vi "Find Version of Installed Driver 2012 NIVerified.vi"() -> ()   [LabVIEW 2012]
uses:
  <vilib>/nisyscfg/Get Installed Components.vi
  <vilib>/nisyscfg/Close (System).vi
  <vilib>/nisyscfg/nisyscfg.lvlib
panel:
  out "NI-IMAQdx version":string
  out "NI-Serial version":string
  # "Overview: This example demonstrates a method of programmatically getting the version of the NI Software, Drivers, and or Devices by utilizing the System Configuration API.\nRequirements: \n1. LabVIEW 2012 ( or compatible)\n2. NI System Configuration 5.3.3 (or compatible)\nInstructions: \n1. Configure which drivers you would like to find the driver version in the block diagram in the two string constants (This example uses NI-IMAQdx and NI-Serial)\n2.\tRun the VI as is or use it as a SubVI in an application\n3.\tObserve the driver version in the string indicators on the front panel"
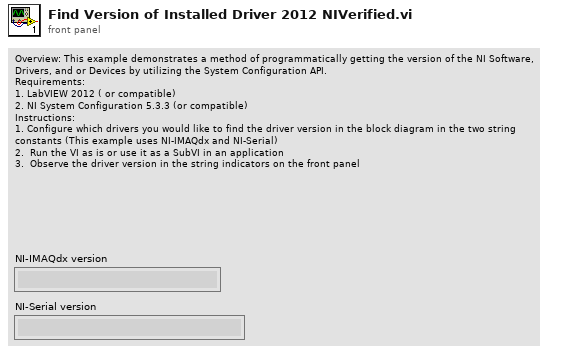
[diagram p1: front panel]
types:
  T1 = typedef "nisyscfg.lvlib/Software 1.2.ctl" = cluster{"title":string, "description":string, "ID":string, "version":string, "component type":T2}
  T2 = typedef "nisyscfg.lvlib/Component Type.ctl" = u32
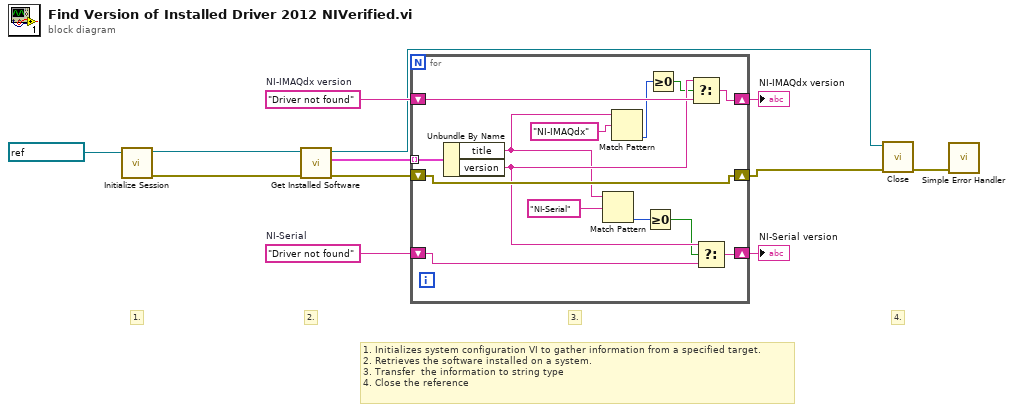
[diagram p0: block diagram]
diagram:
  w10 = "Driver not found"  # NI-Serial
  w11 = "Driver not found"  # NI-IMAQdx version
  # "4."
  # "3."
  # "2."
  # "1. Initializes system configuration VI to gather information from a specified target.\n2. Retrieves the software installed on a system.\n3. Transfer  the information to string type \n4. Close the reference"
  # "1."
  n1 = call <vilib>:"Initialize Session.vi"("Target (localhost)"=refnum<k21> "localhost" ("session in")) -> ("error out"=w5:errorcluster, "Session out"=w6:refnum<k21>)  [unwired: 9 in]
  n2 = call-poly <vilib>:"Get Installed Software.vi"("error in (no error)"=w5, "Session in"=w6) -> ("error out"=w3:errorcluster, "Software Components"=w12:T1[], "Session out"=w4:refnum<k21>)  [unwired: 7 in]
  n3 = for {
    tunnel: w12 -> [w26] mode=indexing
    shift-right: [w24] -> w9
    shift-left: w11 -> [w25]
    shift-right: [w22] -> w8
    shift-left: w10 -> [w23]
    shift-right: [w21] -> w2
    shift-left: w3 -> [w21]
    n4 = Unbundle By Name(w26) -> ("title"=w15:string, "version"=w20:string)
    n5 = Match Pattern(string=w15, regular expression="NI-Serial" ("y")) -> (offset past match=w18:i32)  [unwired: 1 in, 3 out]
    n6 = Match Pattern(string=w15, regular expression="NI-IMAQdx" ("x")) -> (offset past match=w14:i32)  [unwired: 1 in, 3 out]
    n7 = Greater Or Equal To 0?(x=w18) -> (x >= 0?=w17:bool)
    n8 = Greater Or Equal To 0?(x=w14) -> (x >= 0?=w13:bool)
    n9 = Select(t=w20, s=w13, f=w25) -> (s? t:f=w24:string)
    n10 = Select(t=w20, s=w17, f=w23) -> (s? t:f=w22:string)
  }
  "NI-IMAQdx version" <- w9
  "NI-Serial version" <- w8
  n11 = call-poly <vilib>:"Close.vi"("error in (no error)"=w2, "Session in"=w4) -> ("error out"=w1:errorcluster)  [unwired: 9 in]
  n12 = call <vilib>:"Simple Error Handler.vi"("error in (no error)"=w1) -> ()  [unwired: 4 in, 5 out]
